vi "BuildServerTitleText.vi"(3 "ROS":T1={"topic port"=0, "Node"="", "topic"="", "type"="", "node port"=0, "error "={"status"=FALSE, "code"=0, "source"=""}, "Direction"=enum."Node", "Update (ms)"=1, "FIFO size"=0}) -> (0 "text":string, 1 "colored text":string)   [LabVIEW 2014]
doc: "Builds server title for website logs"
uses:
  <userlib>/ROS for LabVIEW Software.lnk/ROS/Code/SubVIs/_ROSControl.ctl
  <userlib>/ROS for LabVIEW Software.lnk/ROS/Code/SubVIs/_ROSDirection.ctl
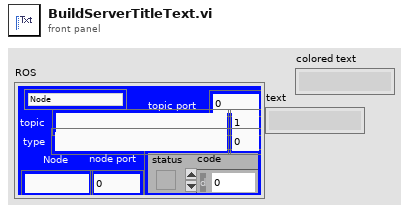
[diagram p1: front panel]
types:
  T1 = typedef "_ROSControl.ctl" = cluster{"topic port":u16, "Node":string, "topic":string, "type":string, "node port":u16, "error ":errorcluster, "Direction":T2, "Update (ms)":u16, "FIFO size":u16}
  T2 = typedef "_ROSDirection.ctl" = enum16{"Node", "Publisher", "Subscriber", "ServiceClient", "ServiceProvider"}
  T3 = enum16{"http://IP:port", "http://IP", "IP:port", "IP only"}
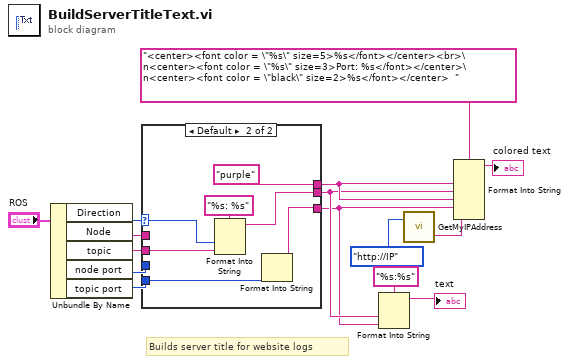
[diagram p0: block diagram]
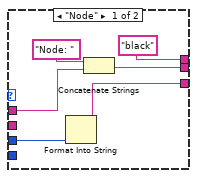
[diagram p2: hidden frame]
diagram:
  # "Builds server title for website logs"
  n1 = Unbundle By Name("ROS") -> ("Direction"=w12:T2, "Node"=w13:string, "topic"=w14:string, "node port"=w8:u16, "topic port"=w7:u16)
  n2 = case shown="Default" w12 {
    selector: w12 -> [_ w27]
    tunnel: w13 -> [w19 _]
    tunnel: w14 -> [_ w26]
    tunnel: [w18 w25] -> w5
    tunnel: ["black" ("format string") "purple" ("format string")] -> w9
    tunnel: w8 -> [w17 _]
    tunnel: [w16 w22] -> w4
    tunnel: w7 -> [_ w23]
    frame "Node" {
      n3 = Format Into String(w17) -> (resulting string=w16:string)  [unwired: 3 in, 1 out]
      n4 = Concatenate Strings("Node: " ("format string"), w19) -> (w18:string)
    }
    frame Default {
      n5 = Format Into String(format string="%s: %s", w27, w26) -> (resulting string=w25:string)  [unwired: 2 in, 1 out]
      n6 = Format Into String(w23) -> (resulting string=w22:string)  [unwired: 3 in, 1 out]
    }
  }
  n7 = Format Into String(format string="%s:%s", w5, w4) -> (resulting string=→"text":string)  [unwired: 2 in, 1 out]
  n8 = call <userlib>:"GetMyIPAddress.vi"("Format"=T3."http://IP") -> ("URI"=w2:string)  [unwired: 1 in, 1 out]
  n9 = Format Into String(format string="<center><font color = \"%s\" size=5>%s</font></center><br>\n<center><font color = \"%s\" size=3>Port: %s</font></center>\n<center><font color = \"black\" size=2>%s</font></center>  " ("string"), w9, w5, w9, w4, w2) -> (resulting string=→"colored text":string)  [unwired: 2 in, 1 out]
